vi "Write Configuration  Data.vi"(8 "error in (no error)":errorcluster, 10 "Configuration Setting":T1={"offset"=0.0, "Signal Type"=enum."Sine Wave", "Amplitude"=1.0, "Frequency"=10.0, "Phase"=0.0, "Noise Amplitude "=1.0} {"Noise Amplitude" format="%.2p"; "Phase" format="%.2p"; "Frequency" format="%0.2p"; "Amplitude" format="%0.2p"; "offset" format="%0.2p"}, 11 "Path":path) -> (0 "error out":errorcluster)   [LabVIEW 2020]
uses:
  <vilib>/Utility/config.llb/Write Key (Double).vi
  <vilib>/Utility/config.llb/Write Key (U32).vi
  <vilib>/Utility/config.llb/NI_LVConfig.lvlib
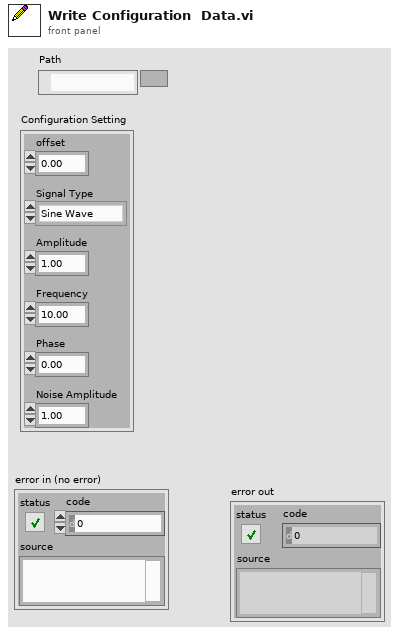
[diagram p1: front panel]
types:
  T1 = cluster{"offset":dbl, "Signal Type":enum16{"Sine Wave", "Triangle Wave", "Square Wave", "Sawtooth Wave"}, "Amplitude":dbl, "Frequency":dbl, "Phase":dbl, "Noise Amplitude ":dbl}
  T2 = enum16{"Sine Wave", "Triangle Wave", "Square Wave", "Sawtooth Wave"}
  T3 = typedef "NI_LVConfig.lvlib/Config Data RefNum.ctl" = refnum<k1>
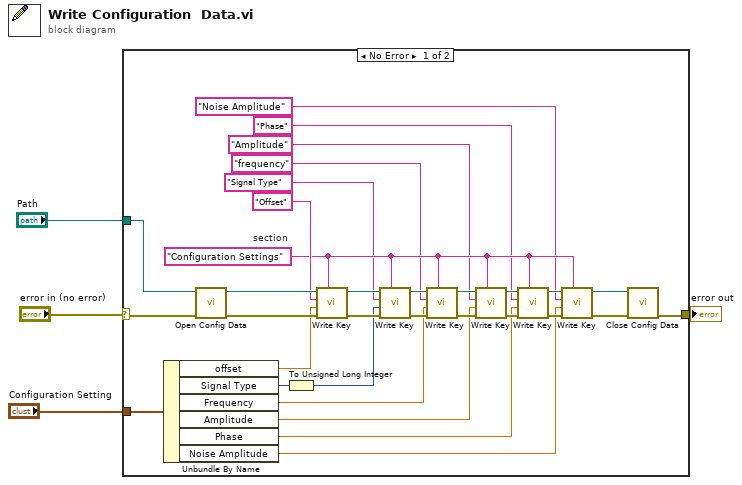
[diagram p0: block diagram]
diagram:
  n1 = case shown="No Error" "error in (no error)" {
    selector: "error in (no error)" -> [w22 w37]
    tunnel: "Configuration Setting" -> [w36 _]
    tunnel: "Path" -> [w23 _]
    tunnel: [w6 w37] -> w1
    frame No Error {
      w20 = "Configuration Settings"  # section
      n2 = Unbundle By Name(w36) -> ("offset"=w14:dbl, "Signal Type"=w13:T2, "Frequency"=w12:dbl, "Amplitude"=w11:dbl, "Phase"=w10:dbl, "Noise Amplitude"=w9:dbl)
      n3 = call <vilib>:"Open Config Data.vi"("error in (no error)"=w22, "configuration file path"=w23) -> ("error out"=w35:errorcluster, "refnum"=w34:T3)  [unwired: 7 in, 1 out]
      n4 = To Unsigned Long Integer(number=w13) -> (unsigned 32bit integer=w5:u32)
      n5 = call-poly <vilib>:"Write Key.vi"("section"=w20, "error in (no error)"=w35, "value"=w14, "key"="Offset" ("section"), "refnum"=w34) -> ("error out"=w33:errorcluster, "refnum out"=w32:T3)  [unwired: 4 in, 1 out]
      n6 = call-poly <vilib>:"Write Key.vi"("section"=w20, "error in (no error)"=w33, "value"=w5, "key"="Signal Type" ("section"), "refnum"=w32) -> ("error out"=w31:errorcluster, "refnum out"=w30:T3)  [unwired: 4 in, 1 out]
      n7 = call-poly <vilib>:"Write Key.vi"("section"=w20, "error in (no error)"=w31, "value"=w12, "key"="frequency" ("section"), "refnum"=w30) -> ("error out"=w29:errorcluster, "refnum out"=w28:T3)  [unwired: 4 in, 1 out]
      n8 = call-poly <vilib>:"Write Key.vi"("section"=w20, "error in (no error)"=w29, "value"=w11, "key"="Amplitude" ("section"), "refnum"=w28) -> ("error out"=w27:errorcluster, "refnum out"=w26:T3)  [unwired: 4 in, 1 out]
      n9 = call-poly <vilib>:"Write Key.vi"("section"=w20, "error in (no error)"=w27, "value"=w10, "key"="Phase" ("section"), "refnum"=w26) -> ("error out"=w25:errorcluster, "refnum out"=w24:T3)  [unwired: 4 in, 1 out]
      n10 = call-poly <vilib>:"Write Key.vi"("section"=w20, "error in (no error)"=w25, "value"=w9, "key"="Noise Amplitude" ("section"), "refnum"=w24) -> ("error out"=w7:errorcluster, "refnum out"=w8:T3)  [unwired: 4 in, 1 out]
      n11 = call <vilib>:"Close Config Data.vi"("error in (no error)"=w7, "refnum"=w8) -> ("error out"=w6:errorcluster)  [unwired: 8 in, 1 out]
    }
    frame Error {
    }
  }
  "error out" <- w1
